vi "2020_day04.vi"() -> ()   [LabVIEW 2021]
uses:
  <vilib>/regexp/Match Regular Expression.xnode
panel:
  out "Task 2":i16
  out "Task 1":i16
  in  "Switch":bool caption="Ex. Data  vs.  User Data"
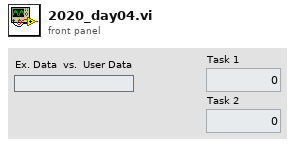
[diagram p1: front panel]
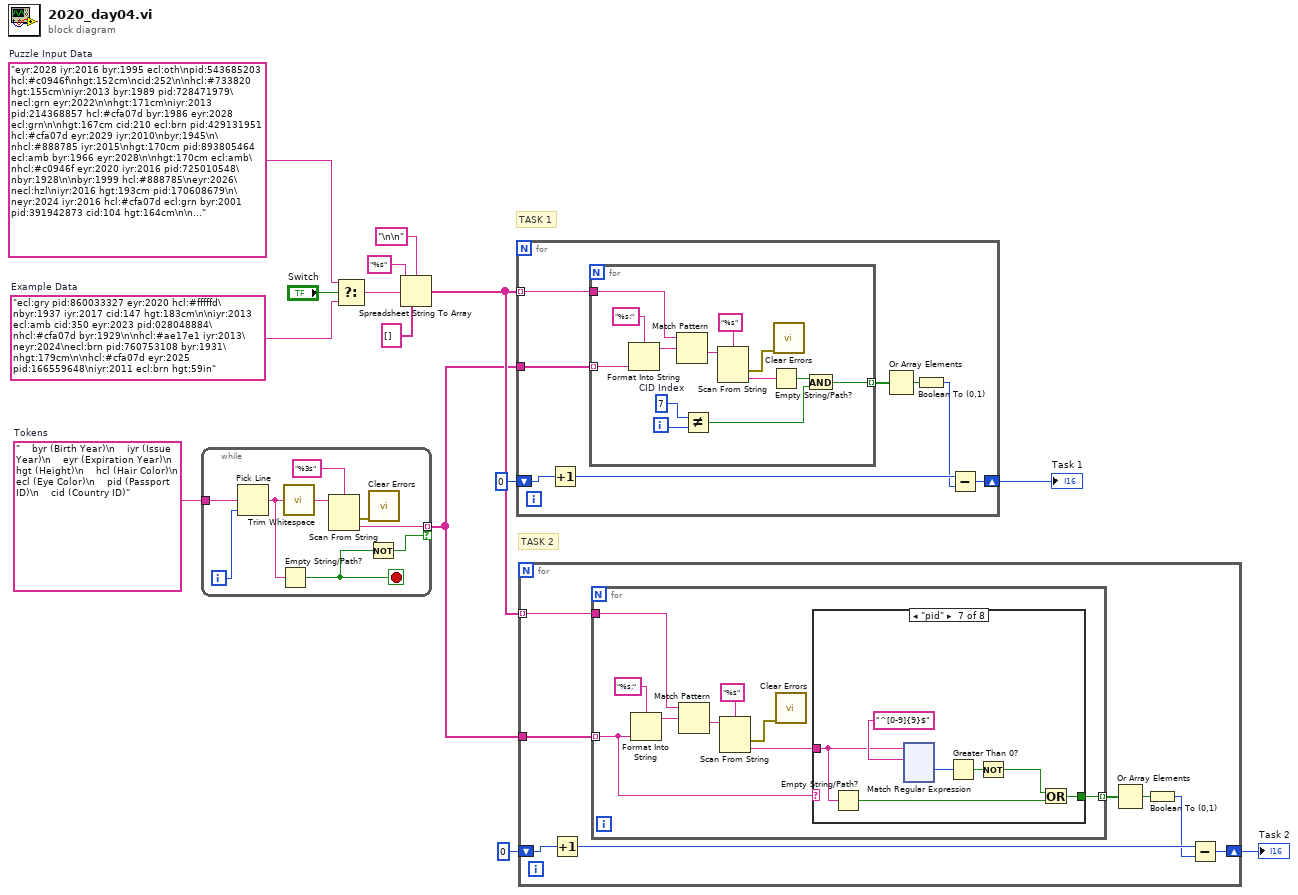
[diagram p0: block diagram]
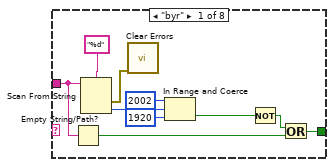
[diagram p2: hidden frame]
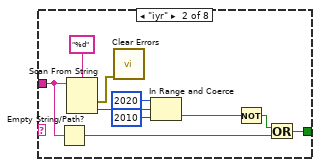
[diagram p3: hidden frame]
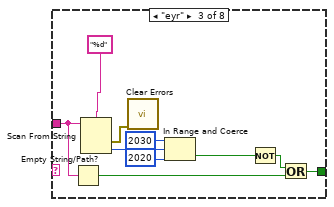
[diagram p4: hidden frame]
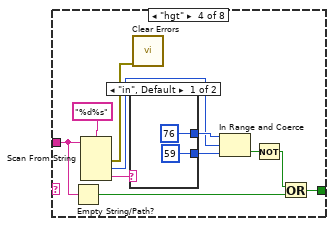
[diagram p5: hidden frame]
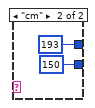
[diagram p6: hidden frame]
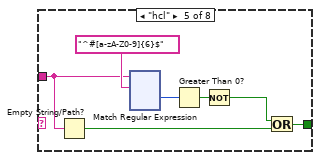
[diagram p7: hidden frame]
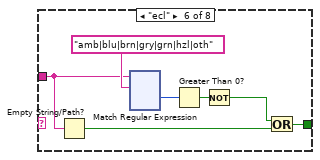
[diagram p8: hidden frame]
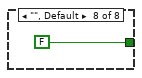
[diagram p9: hidden frame]
diagram:
  w7 = "    byr (Birth Year)\n    iyr (Issue Year)\n    eyr (Expiration Year)\n    hgt (Height)\n    hcl (Hair Color)\n    ecl (Eye Color)\n    pid (Passport ID)\n    cid (Country ID)"  # Tokens
  w12 = "eyr:2028 iyr:2016 byr:1995 ecl:oth\npid:543685203 hcl:#c0946f\nhgt:152cm\ncid:252\n\nhcl:#733820 hgt:155cm\niyr:2013 byr:1989 pid:728471979\necl:grn eyr:2022\n\nhgt:171cm\niyr:2013 pid:214368857 hcl:#cfa07d byr:1986 eyr:2028 ecl:grn\n\nhgt:167cm cid:210 ecl:brn pid:429131951 hcl:#cfa07d eyr:2029 iyr:2010\nbyr:1945\n\nhcl:#888785 iyr:2015\nhgt:170cm pid:893805464 ecl:amb byr:1966 eyr:2028\n\nhgt:170cm ecl:amb\nhcl:#c0946f eyr:2020 iyr:2016 pid:725010548\nbyr:1928\n\nbyr:1999 hcl:#888785\neyr:2026\necl:hzl\niyr:2016 hgt:193cm pid:170608679\n\neyr:2024 iyr:2016 hcl:#cfa07d ecl:grn byr:2001 pid:391942873 cid:104 hgt:164cm\n\niyr:2019\neyr:2025 pid:138912840 byr:1996\nhgt:166cm\nhcl:#888785 ecl:grn\n\niyr:2023 hcl:a58381 pid:#401a29 eyr:1940\nbyr:1920\necl:utc hgt:183cm\n\npid:493510244 ecl:gry hgt:153cm byr:1950 cid:181 eyr:2028\nhcl:#ceb3a1\niyr:2020\n\niyr:2018 pid:074340974 hgt:182cm\nhcl:#866857 byr:1988 ecl:hzl eyr:2023\n\nhcl:#866857 ecl:oth byr:1977 iyr:2014 hgt:180cm pid:860745884\neyr:2023\n\neyr:2026 pid:815594641\necl:gry iyr:2012 byr:1992 hgt:161cm hcl:#b6652a\n\necl:gry cid:338 eyr:2021 pid:777099878 hgt:193cm hcl:#efcc98\nbyr:1945\niyr:2015\n\niyr:2016 byr:1934 hcl:#b6652a\nhgt:162cm ecl:hzl\ncid:296\npid:742610207\neyr:2022\n\necl:#ba3242\nhgt:80 byr:1931\npid:550004054 iyr:1949 eyr:1944 hcl:fb3859\n\necl:amb eyr:2024\nbyr:1965 iyr:2010 pid:094059049\nhcl:#fffffd\nhgt:168cm\n\npid:159cm\niyr:1923 eyr:2032 hcl:701107 cid:343 ecl:gmt byr:2010\nhgt:177cm\n\neyr:2021\necl:grn byr:1991\nhcl:#fffffd hgt:167cm pid:243218792 iyr:2019\n\nhgt:157cm byr:2017 ecl:grn iyr:2012\neyr:2030 hcl:#18171d pid:173cm\n\npid:260101979 hgt:187cm eyr:2033 ecl:lzr\nbyr:2020 hcl:1058ce cid:133 iyr:2012\n\nhcl:#7d3b0c\npid:307828343 byr:2001\ncid:317 iyr:2013\neyr:2029\n\npid:472940417 eyr:1960\nhgt:181cm hcl:#c0946f cid:269\nbyr:2014\niyr:1956\n\nhcl:#18171d eyr:2021 byr:2001 pid:421443124\necl:brn iyr:2020 hgt:156cm\n\ncid:347 hgt:60in pid:359783692 byr:1932\necl:hzl\neyr:2023\nhcl:#888785 iyr:2019\n\npid:230915137\nbyr:1999\niyr:2011 eyr:2020 hcl:#7d3b0c ecl:hzl\nhgt:164cm\n\niyr:1989\nbyr:2008\nhgt:154cm\neyr:2028 pid:280298169\ncid:208\necl:oth\n\nbyr:1954 iyr:2017\necl:hzl\neyr:2026\npid:966957581 hgt:175cm hcl:#18171d\n\npid:308053355 hgt:192cm eyr:2022 ecl:amb cid:146 iyr:2015\nbyr:1991 hcl:#c0946f\n\nhcl:#a97842 pid:244441133 iyr:2019\nhgt:182cm\necl:amb cid:172 byr:1973 eyr:2029\n\niyr:2017\nbyr:1985 cid:215\necl:blu hcl:#623a2f hgt:160cm pid:157856689 eyr:2030\n\neyr:2027 ecl:#d72f9b hgt:162cm\niyr:2018 hcl:#a97842\nbyr:1945\npid:131243258\n\nhcl:#b3f2f0 pid:204254353 cid:169 eyr:2020\niyr:2013 hgt:172cm ecl:blu byr:1950\n\nbyr:1957 hcl:#c0946f hgt:152cm ecl:blu eyr:2027 pid:325917033\niyr:2010\n\necl:oth byr:1950 hgt:166cm pid:007352351\nhcl:#b6652a\niyr:2020\neyr:2024\n\nhgt:165 eyr:2030 iyr:2027\necl:#1a34f1 pid:2894591864 byr:2024 hcl:z\n\nbyr:1971 ecl:oth\nhgt:163cm eyr:2021 pid:040443396\n\nhgt:177cm\nbyr:1955 pid:585735590 iyr:2010 ecl:grn eyr:2024\nhcl:#602927\n\ncid:74\niyr:2010\npid:014378493 hgt:174cm eyr:2020\necl:grn byr:1944\n\npid:404141049\nbyr:1947 ecl:blu hgt:170cm iyr:2011\neyr:2028\nhcl:#cfa07d\n\necl:hzl byr:1938 pid:235085606 cid:180 hcl:8fb74c eyr:2021 hgt:73 iyr:2015\n\npid:860077423 ecl:gry\nhcl:#3e845b\nhgt:167cm byr:1933 iyr:2016 eyr:2021\n\nhcl:#733820 hgt:66in eyr:1920\necl:oth byr:1941 pid:979460474 iyr:2010\ncid:247\n\nhcl:#cfa07d ecl:#13bd36 hgt:193cm eyr:2027 pid:181cm byr:1952 iyr:1951\n\necl:brn hcl:#602927\nhgt:161cm\neyr:2027 pid:822749462 byr:1946\niyr:2014\n\nbyr:2013\niyr:2021 ecl:zzz eyr:2032 hgt:193in hcl:#a97842 pid:163cm\n\neyr:2029 cid:140\nbyr:1984\niyr:2018 hgt:187cm hcl:#b6652a pid:910674579\n\necl:hzl hgt:173cm pid:096026282\niyr:2014 byr:1956\neyr:2029 hcl:#866857\n\neyr:2024 iyr:2019 pid:301205967\ncid:276 byr:1957 hcl:#3fec29 ecl:gry hgt:165cm\n\niyr:2013 ecl:oth hgt:177cm hcl:#6b5442 eyr:2021 byr:1962 pid:006347857\n\necl:grt byr:1983 hcl:#cfa07d\nhgt:163cm\neyr:1979\niyr:1958 pid:796395720\n\niyr:2011 pid:415403544 hcl:#c0946f byr:1990 ecl:oth eyr:2023 hgt:73in\ncid:107\n\nhgt:166cm eyr:2029 iyr:2015\nhcl:#c0946f ecl:brn\nbyr:1964\npid:469449137\n\neyr:2023\nbyr:1969 iyr:2010 hgt:163cm hcl:#a97842 pid:570942274\necl:blu\n\nhcl:#623a2f\necl:brn hgt:183cm pid:524675399\neyr:2020 iyr:2012 byr:1981\n\niyr:2017 hcl:#fffffd eyr:2026\necl:gry byr:1979 hgt:152cm pid:505790864\n\nhgt:68in\nhcl:#c0946f iyr:2012\neyr:2023 pid:933562997 byr:1993\necl:grn\n\npid:267705171\nhgt:166cm byr:1970 iyr:2019 hcl:#341e13 ecl:oth\neyr:2030\n\necl:brn byr:1972 eyr:2026 pid:774637408 hgt:189cm iyr:2015 hcl:#341e13\n\nhgt:175cm eyr:2026 byr:2001 iyr:2020\nhcl:#733820 ecl:blu pid:686996160\n\nhgt:190cm hcl:#c0946f pid:228444464 byr:1987\niyr:2020 eyr:2030\necl:blu\n\nbyr:1990 hgt:179cm\npid:885359438 eyr:2028 iyr:2010 ecl:amb\nhcl:#67067e\n\nbyr:1945 hcl:#866857 eyr:2022 iyr:2019\npid:708146656 cid:65\nhgt:172cm ecl:brn\n\necl:hzl hgt:191cm\ncid:260 pid:010716679 iyr:2011 eyr:2029 byr:1920 hcl:#efcc98\n\niyr:2012\ncid:313 pid:264894705 byr:1951 hcl:#733820 eyr:2030 ecl:blu\nhgt:178cm\n\neyr:2027 pid:790510379\niyr:2013\necl:amb\nhgt:186cm\nhcl:#866857\nbyr:1926\n\npid:535750794 hgt:191cm iyr:2016 hcl:#a97842 eyr:2029\necl:hzl byr:1923\n\nbyr:2023 pid:#eb4c2a iyr:1939 ecl:grn hcl:06d729 hgt:73 eyr:2038\n\npid:792365221 iyr:2013 ecl:oth\nbyr:1997\nhgt:170cm hcl:#efcc98\neyr:2022\n\nhgt:192cm pid:874141668\nbyr:1957 iyr:2015\necl:gry\n\nhcl:#b6652a pid:770238761 eyr:2029 byr:1934 iyr:2013\necl:blu cid:177\nhgt:184cm\n\necl:hzl eyr:2024 hgt:72in pid:546439165\niyr:2013\nhcl:#c0946f cid:223 byr:1989\n\nbyr:1985\necl:utc pid:#ff1cbf\niyr:2018 hcl:#866857 hgt:169cm eyr:2026 cid:194\n\nhgt:189cm\neyr:2026 pid:120642045 ecl:blu\nhcl:#602927 cid:177\nbyr:1954 iyr:2012\n\npid:314624973\nbyr:1959 iyr:2015 hcl:#c0946f ecl:grn\neyr:2027 cid:349 hgt:156cm\n\nbyr:1978\niyr:2020 hgt:150cm cid:266 eyr:2026\npid:443912835 hcl:#b6652a\n\nhgt:174cm byr:1974 pid:729198828\necl:brn iyr:2014\nhcl:#18171d eyr:2027\n\npid:472891001 ecl:xry\nhgt:96 hcl:1b816a iyr:1954\nbyr:2015 eyr:2037\n\nbyr:1966 eyr:2022\niyr:2014\npid:848187688 hcl:#602927 ecl:gry hgt:152cm\n\nhgt:129 eyr:2037 cid:61 iyr:2009 byr:2027 hcl:#c0946f\npid:3569865\necl:#4e3d72\n\necl:gry\neyr:2021 pid:234525998 byr:1964 hgt:168cm cid:140\nhcl:#7d3b0c iyr:2013\n\necl:xry\ncid:86\nhgt:172in\nbyr:1972\niyr:2015 hcl:#7d3b0c pid:833809421 eyr:2030\n\npid:444365280 hgt:72in\necl:brn\nhcl:#b6652a byr:1985 eyr:2027 iyr:2012\n\niyr:2010 byr:2013 hgt:181cm eyr:2021\npid:072317444\necl:oth hcl:#866857\ncid:118\n\npid:4354408888 iyr:2012\nhcl:#b6652a cid:104\nhgt:96 eyr:2020\nbyr:1933 ecl:amb\n\neyr:2023 ecl:gry hcl:#a97842 pid:287719484 byr:1994\niyr:2011 hgt:163cm cid:299\n\nbyr:1932\nhgt:170cm\niyr:2014 pid:777844412 eyr:2040 hcl:#cfa07d ecl:brn\n\ncid:160 hgt:191cm eyr:2020 iyr:2012\necl:brn byr:1981 pid:077027782\n\ncid:182 hgt:176cm hcl:#7d3b0c\neyr:2030 ecl:blu pid:096742425 iyr:2010 byr:1963\n\nbyr:2010 cid:337 hcl:z pid:525126586 iyr:2010 hgt:73cm eyr:2040 ecl:blu\n\necl:gry\niyr:2017\nhgt:185cm hcl:#6b5442 byr:1993\neyr:2029 pid:366083139 cid:343\n\neyr:2028 ecl:amb\npid:878658841 byr:1960 hgt:179cm hcl:#18171d iyr:2010\n\npid:537309261 iyr:2015 hgt:187cm\nhcl:#4fe831 eyr:2026\necl:blu byr:1982\n\necl:brn hgt:163cm\neyr:2021 hcl:#6b5442 byr:1979 iyr:2013 pid:924759517\n\npid:683651053 hcl:#179c55\necl:blu byr:1989 hgt:190cm\niyr:2016\neyr:2030\n\necl:grn\niyr:2016 hcl:#b6652a\nbyr:1994 eyr:2020 pid:448424292 hgt:174cm\n\nhgt:157cm\necl:grn\nbyr:2000\npid:734707993 hcl:#341e13 iyr:2020\n\nhcl:#341e13 hgt:156cm iyr:2020 pid:299213638\nbyr:1947 ecl:hzl eyr:2023\n\nhgt:193cm hcl:#b6652a iyr:2014 ecl:hzl byr:1947 eyr:2025\npid:044486467\n\nbyr:1975\nhgt:159cm\necl:grn pid:318489576 eyr:2029 hcl:#6b5442\niyr:2020\n\niyr:2018 pid:512971930\nhcl:#888785 byr:1966 eyr:2024 hgt:158cm\ncid:100 ecl:gry\n\necl:amb eyr:2030 hgt:171cm hcl:#efcc98 pid:800921581 cid:339 byr:1980 iyr:2017\n\niyr:2019 cid:172\nhgt:152cm\neyr:2022 ecl:oth hcl:#602927 byr:1960\n\niyr:2019 pid:762312913\neyr:2029\necl:hzl\nhcl:#6b5442\nbyr:1940\nhgt:169cm cid:289\n\neyr:2022 ecl:gry byr:1976\niyr:2020 hcl:#733820 hgt:172cm pid:040331561\n\nhgt:171cm ecl:brn iyr:2013 eyr:2027 byr:1940 hcl:#a6e32a pid:223986941\n\nhcl:#341e13\neyr:2028 ecl:amb byr:1942\nhgt:166cm pid:435382099 iyr:2020\n\ncid:298 pid:641326891\nhgt:155cm hcl:#623a2f ecl:grn byr:1981 eyr:2025\niyr:2010\n\niyr:2015 pid:472000322 eyr:2021 byr:1977\necl:gry hgt:165cm cid:270\n\neyr:2027 byr:1956\npid:193087729 hcl:#ceb3a1\ncid:213 hgt:193cm ecl:oth\n\niyr:2014\nbyr:1971 cid:96\nhgt:74in\npid:136003336\neyr:2020 ecl:hzl hcl:#efcc98\n\nhcl:z pid:097595072 ecl:amb\niyr:2015 byr:2021\neyr:2039 hgt:188cm\n\npid:74823273\nhcl:#341e13\ncid:166 hgt:182cm byr:2026 iyr:2027 ecl:amb\neyr:2032\n\nbyr:1932 eyr:2022 pid:367248062 hgt:182cm ecl:oth hcl:#c0946f\niyr:2020\n\nhgt:72cm\niyr:2015 cid:234 byr:2013\necl:brn pid:9401866358\n\npid:022399779 iyr:2010 byr:1969 hcl:#6b5442\necl:grn eyr:2020\nhgt:189cm\n\nbyr:1971 iyr:2011 cid:161 ecl:brn hgt:153cm\neyr:2028 pid:819137905 hcl:#cfa07d\n\ncid:161 hgt:159cm iyr:2011 pid:815860793 hcl:#a97842 ecl:grn byr:1972 eyr:2027\n\necl:amb\nhgt:118 byr:1981 iyr:2019\nhcl:#a97842 eyr:2021 pid:270790642\n\nhcl:#b6652a pid:732272914 eyr:2030 hgt:183cm ecl:hzl\nbyr:1934\niyr:2018\n\neyr:2027\npid:877388498 hcl:#ceb3a1\nbyr:1925 cid:236 ecl:grn\niyr:2019 hgt:191cm\n\neyr:2020 ecl:brn hcl:#fffffd hgt:181cm pid:801311341 byr:1986 iyr:2010\n\nbyr:1925 cid:179 ecl:hzl pid:360641953 eyr:2030\nhgt:171in iyr:2015\nhcl:#602927\n\ncid:83 hgt:181cm\neyr:2028 byr:1941 pid:165937945 hcl:#888785 iyr:2014\necl:grn\n\nhcl:#a97842 byr:1928\niyr:2013\npid:870072019 hgt:76in\necl:oth cid:127 eyr:2026\n\ncid:169\nhgt:187cm pid:008180128 iyr:2013 byr:1991 hcl:#7d3b0c ecl:hzl eyr:2026\n\necl:amb\neyr:2027 hgt:155cm pid:586151564 iyr:2010\nbyr:1949\nhcl:#18171d\n\nhgt:167cm\niyr:2010 byr:1982 ecl:amb\ncid:235 pid:557737957 eyr:2020\nhcl:#ceb3a1\n\necl:grn byr:1939 hcl:#733820\neyr:2026 pid:993218958 iyr:2010\nhgt:150cm\n\nhgt:68in ecl:blu\nbyr:1965 iyr:2017 pid:854858050 eyr:2021\n\necl:gry pid:347763159 eyr:2024 iyr:2017 byr:1961\nhgt:151cm\nhcl:#623a2f\n\necl:utc hcl:#602927\npid:#1408ff byr:1941\ncid:82\niyr:2015 hgt:185cm eyr:2028\n\niyr:2020 hgt:151cm eyr:2025\nbyr:1934 hcl:#888785\npid:396545094 ecl:oth\n\nhgt:153cm\neyr:2028 hcl:#733820 ecl:gry iyr:2019\npid:081352630 byr:1943\n\neyr:2030\niyr:2011\necl:grn pid:313741119\nhgt:161cm byr:1946\nhcl:#a97842\n\nbyr:1968 ecl:gry\npid:742357550\neyr:2024 hcl:#18171d iyr:2018\nhgt:157cm\n\npid:387505919\necl:oth byr:1945\niyr:2014\nhgt:190cm hcl:#888785\neyr:2028\n\niyr:2017 hgt:175cm\nbyr:1989 eyr:2022\nhcl:#b6652a pid:499016802 ecl:gry cid:136\n\npid:490807331 iyr:2016\nhcl:#ceb3a1\nhgt:150cm eyr:2026\necl:amb byr:1967\n\niyr:2011\nhgt:155in\nhcl:#ceb3a1 pid:118497416\neyr:2029 byr:2011 ecl:oth\n\nhcl:03a888 byr:2029\necl:#6f7292 eyr:1969 iyr:2028 hgt:162cm pid:73551266\n\niyr:2016 hgt:182cm\nbyr:1966 ecl:grn eyr:2022\nhcl:#fffffd pid:061720787\n\nbyr:1971 hcl:z\neyr:2035 pid:158cm\necl:#d3ec19\n\nhcl:#623a2f hgt:156cm eyr:2028\necl:brn iyr:2013\nbyr:1980 pid:112283719\n\neyr:2020\nbyr:1956 iyr:2013\nhcl:#6b5442\necl:grn pid:876589775 hgt:179cm\n\nhgt:138\nbyr:2013 eyr:2040 iyr:2028 cid:197 ecl:#8844fd pid:8524414485\nhcl:z\n\neyr:2040\nhgt:173in hcl:z pid:#654654 byr:2016 iyr:2022 ecl:#452d22\n\niyr:2012 cid:265 eyr:2021 hgt:192cm\nbyr:1993 ecl:brn\n\neyr:2026 hcl:#888785\nhgt:158cm byr:1942\niyr:2015\necl:amb pid:546984106\n\niyr:2019\necl:hzl\nbyr:1922 eyr:2028 hgt:172cm\npid:465052232 hcl:#602927\n\npid:710362693 eyr:2023\nhcl:#c0946f byr:1951 ecl:grn\niyr:2019 hgt:190cm\n\niyr:2024 pid:#a08e69\nhcl:z byr:1966 ecl:#7b9978 eyr:2035\nhgt:69cm\n\nhcl:#efcc98\npid:164cm\niyr:2010 cid:194 hgt:71cm byr:1923 eyr:2026\n\nhgt:65in\niyr:2019 byr:1969 pid:466669360 eyr:2022 ecl:brn hcl:#b6652a\n\npid:42472559 hcl:#6f5763\neyr:2035\niyr:2014 hgt:154in byr:1939 ecl:grt cid:323\n\npid:715680334 hgt:166cm cid:283\nbyr:1982\niyr:2015 eyr:2030 hcl:#ceb3a1 ecl:grn\n\neyr:2018 iyr:2029\necl:brn\nbyr:2022 pid:#ff6df1\nhcl:z\nhgt:68cm\n\npid:094541122\neyr:2024 byr:1940\necl:amb iyr:2019 hgt:64in hcl:#733820\n\nhgt:163in\neyr:2022 ecl:utc hcl:#ceb3a1 iyr:2028\n\necl:gry pid:53552934\nhgt:193 byr:2021\neyr:2028\niyr:2011 cid:98 hcl:90c63f\n\neyr:2024 hcl:#cfa07d ecl:brn\niyr:2019 byr:1993 hgt:156cm pid:449484188\n\niyr:2020\nhgt:164cm hcl:#623a2f\npid:820731743 eyr:2025\nbyr:1997 ecl:hzl\n\nhcl:47242b ecl:utc hgt:156\npid:#9a9903 eyr:2030 iyr:1990\nbyr:2011\n\nhcl:#602927\nhgt:189cm\npid:949021883 iyr:2014 ecl:oth cid:327\neyr:2027 byr:1953\n\nhgt:189cm cid:301\nbyr:1982\necl:grn\neyr:2028 hcl:#733820 pid:796040143 iyr:2015\n\ncid:169 iyr:2013 pid:355177646 byr:1988\necl:oth\nhcl:#cfa07d\nhgt:185cm eyr:2022\n\npid:563150261 eyr:2020 ecl:brn byr:1996 hcl:#7d3b0c iyr:2018 hgt:189cm cid:84\n\ncid:188 eyr:2027\nbyr:1944\npid:486184923\niyr:2010 hgt:193cm hcl:#341e13 ecl:oth\n\niyr:2019\nbyr:1969 hgt:152cm pid:430698432 ecl:gry hcl:#888785 eyr:2026 cid:293\n\necl:gry\ncid:270 hcl:#602927 iyr:2017 hgt:151cm eyr:2029 pid:051398739 byr:1954\n\necl:oth eyr:2030 pid:024655030\nhgt:184cm byr:1969\nhcl:#18171d\n\neyr:2030\npid:899973263 hgt:178cm byr:1987 hcl:#cfa07d iyr:2012\necl:amb\n\niyr:1958 hgt:165cm pid:377677319\necl:grt eyr:2032 byr:2025\nhcl:bbfbe2\n\necl:blu\niyr:2016\nhgt:152cm byr:1964\nhcl:#c4f777\neyr:2021\npid:044307549 cid:80\n\necl:brn pid:330836320\nbyr:1963 cid:217 hgt:169cm\neyr:2024\niyr:2019 hcl:#ceb3a1\n\nbyr:1976 eyr:2027\npid:452662874 hgt:192cm ecl:oth iyr:2018 hcl:#602927\n\neyr:2027 hgt:183cm ecl:brn iyr:2017 hcl:#341e13 pid:827463598\n\necl:brn pid:930667228 cid:310 iyr:2020\neyr:2027 hgt:160cm byr:1932 hcl:#c0946f\n\npid:955804028 byr:1983\nhcl:#fffffd\nhgt:178cm iyr:2013\neyr:2021 ecl:gry\n\nhgt:189cm eyr:2021 pid:430243363 iyr:2015 hcl:#ceb3a1\nbyr:2000 ecl:oth cid:284\n\npid:436671537 hcl:#cfa07d iyr:2011 cid:106 hgt:171cm\necl:blu eyr:2021 byr:1943\n\neyr:2028 hgt:169cm\niyr:2015 pid:177443573 byr:1945\nhcl:#c0946f ecl:gry\n\nhcl:#fffffd byr:1995 eyr:2021\necl:grn\nhgt:192cm iyr:2010 pid:754912745\n\npid:330882171 iyr:2015 cid:211 ecl:grn byr:1961 eyr:2021 hcl:z\nhgt:169cm\n\nbyr:1926 eyr:2029 pid:178633665 cid:141 iyr:2017 hcl:#b99eb9\nhgt:178cm ecl:brn\n\neyr:2022 ecl:hzl hcl:#cfa07d hgt:168cm iyr:2015\nbyr:1982 pid:645675448\n\necl:blu byr:1980 hgt:186cm iyr:2010 cid:94 hcl:#c0946f eyr:2027 pid:384440210\n\ncid:309 hcl:#602927 hgt:192cm eyr:2027 ecl:amb\npid:527932745 iyr:2012 byr:1982\n\ncid:132\necl:blu iyr:2016\neyr:2027 byr:1940 hcl:#341e13 hgt:166cm pid:613386501\n\npid:360563823 eyr:2028 byr:1990 iyr:2016\necl:blu cid:287 hgt:162cm hcl:#888785\n\nhgt:161cm\nbyr:2002\nhcl:#623a2f pid:535361632\necl:gry eyr:2021 iyr:2013\n\nhgt:67in\nbyr:1967\ncid:333 hcl:#cfa07d\niyr:2012 eyr:2024 ecl:hzl pid:538161833\n\necl:#2bc145 eyr:1963 iyr:2030\ncid:241 hcl:2fc384 hgt:156in pid:2899917140\nbyr:2005\n\neyr:2021 pid:021590229 ecl:gry\nhgt:164cm iyr:2013 hcl:#efcc98 byr:1985\n\necl:hzl byr:1943\ncid:279 pid:979130395\niyr:2011\nhgt:165cm\neyr:2021\nhcl:#f331b3\n\nhgt:161cm\nhcl:#888785 byr:1981 pid:835477382 eyr:2025 iyr:2012\ncid:348\necl:blu\n\nhgt:159cm hcl:b4ce6a cid:319 eyr:2035 iyr:1965 ecl:oth\nbyr:2010 pid:158cm\n\niyr:2020\neyr:2026 ecl:grn hcl:#a97842 pid:126915503\nhgt:178cm byr:1986\n\nhgt:184cm ecl:hzl\ncid:67 iyr:2020 eyr:2026 pid:168775568 byr:1944 hcl:#a97842\n\nhcl:#fffffd iyr:2016 pid:379463363\necl:oth\nhgt:179cm byr:1988\neyr:2028\n\nhcl:#cfa07d ecl:amb eyr:2030 pid:320360020\niyr:2016 hgt:172cm byr:1961\n\ncid:221 hcl:#cfa07d byr:1946 eyr:2024 ecl:oth pid:066950409 hgt:173cm\niyr:2020\n\nhcl:#602927 eyr:2028 ecl:gry iyr:2019 pid:583204134 byr:1966 hgt:178cm\n\nbyr:1930\niyr:2020 ecl:hzl\nhcl:#ceb3a1 pid:285751767 cid:287 eyr:2023 hgt:192cm\n\neyr:2024\necl:hzl cid:87 iyr:2015\nhgt:152cm hcl:#18171d pid:959574669\nbyr:1990\n\npid:45938863\nhcl:49c7ce cid:349 hgt:181cm\neyr:2023 ecl:grn iyr:2015 byr:1948\n\nhcl:#866857 iyr:2012 ecl:amb cid:132 byr:1955 hgt:162cm pid:597748286 eyr:2023\n\npid:293364535 byr:2024\nhgt:177cm eyr:2039\niyr:2020 hcl:#dae928 ecl:hzl\n\npid:212659709 iyr:2018\nhgt:188cm\nhcl:#efcc98 byr:1974 eyr:2029 ecl:oth cid:244\n\ncid:140\necl:amb\neyr:2022 hgt:181cm hcl:#efcc98\nbyr:1943\niyr:2016\n\ncid:71 hgt:151cm pid:5063555219 eyr:2023 ecl:hzl\nbyr:2019\nhcl:#7d3b0c iyr:2023\n\nhgt:157in pid:#298b06 iyr:2030 ecl:#66a631 eyr:2035 hcl:z byr:2019\n\nhgt:190cm iyr:1943\npid:644021656 hcl:#6b621c\necl:oth eyr:2021 byr:1923\n\necl:hzl iyr:2012 eyr:2023 pid:881271720 hcl:#ceb3a1 hgt:172cm\nbyr:1957\n\niyr:2017 hcl:#888785\necl:amb hgt:170cm byr:1967 pid:198856675 eyr:2027\n\neyr:2026\necl:gry\npid:834980363 hcl:#733820 byr:1930\nhgt:175cm iyr:2018\ncid:214\n\nhcl:#efcc98 eyr:2029 iyr:2010 pid:980087545\necl:brn hgt:157cm\n\npid:57513658 iyr:2011 byr:1993 ecl:brn eyr:2027 hcl:#6b5442 hgt:165cm\n\necl:hzl\neyr:2025\nhcl:#733820\nhgt:169cm iyr:2018 cid:328 byr:1999 pid:694719489\n\neyr:2023\ncid:125 byr:1925\nhgt:185cm pid:806769540 iyr:2013 ecl:hzl\nhcl:#866857\n\niyr:2010 cid:225\necl:hzl eyr:2027 pid:615545523\nhcl:#733820\nbyr:1994\nhgt:166cm\n\nbyr:1941 ecl:gry iyr:2019 eyr:2026 hgt:73cm hcl:#602927\npid:352996721\n\npid:140250433\neyr:2030 ecl:grn\nhcl:#fffffd iyr:2011 byr:1937 hgt:185cm\n\necl:gry byr:2002 iyr:2017 hcl:#b6652a cid:261 pid:178cm eyr:2022 hgt:166cm\n\necl:grn iyr:2010 eyr:2022 byr:1924\npid:214641920 hcl:#ceb3a1\nhgt:155cm\n\nhcl:z pid:150cm ecl:utc iyr:1981\neyr:2034\nhgt:156in cid:260 byr:2027\n\nbyr:1987 hgt:66in\neyr:2021 pid:876757018 iyr:2015 hcl:d596e4 ecl:hzl\n\ncid:116 ecl:oth hgt:180cm\niyr:2020 byr:1942 hcl:#2fc31f\neyr:2027\npid:253569416\n\npid:509387921\neyr:2022\nhcl:#888785 ecl:oth hgt:193cm\niyr:2012 cid:97\nbyr:1975\n\nhcl:#18171d hgt:190cm pid:062827417 byr:1939\niyr:2019 eyr:2022\necl:hzl\n\niyr:2025\nbyr:2028\nhgt:165in eyr:2027 pid:6259332452\nhcl:#478251\n\niyr:2018 eyr:2026 pid:523863237\nhgt:187cm\necl:oth\nbyr:1944\nhcl:#a97842\n\nhgt:181cm hcl:#733820 pid:923996316\ncid:110\niyr:2011 byr:1949 ecl:blu eyr:2023\n\npid:304792392 hcl:487823 eyr:2020\nhgt:70cm byr:2024\niyr:1953\necl:blu\n\npid:142200694\necl:oth hcl:#888785 eyr:2028\nhgt:152cm byr:1954 iyr:2018\n\necl:utc\niyr:2015 byr:1932 hcl:#623a2f\neyr:2027 hgt:183cm pid:036300444\n\niyr:2014 ecl:hzl byr:1935 hgt:190cm hcl:#efcc98 pid:945893288\neyr:2025\n\nhcl:#efcc98 pid:252639104 hgt:188cm\nbyr:1998 iyr:2019 ecl:grn\neyr:2023\n\nhcl:58aa4a byr:1930 hgt:193cm\niyr:1998 cid:196 ecl:brn\neyr:2032\n\niyr:2015 ecl:hzl\nhgt:193cm pid:653794674 eyr:2024\nhcl:#fffffd byr:1921\n\npid:980680460 byr:1962 ecl:blu\niyr:2013\nhcl:#72cace\neyr:2030\nhgt:180cm\n\neyr:2025\nhgt:182cm hcl:#ceb3a1 iyr:2010 byr:1945 cid:314 pid:597769706 ecl:amb\n\npid:761757504\nhcl:#888785 hgt:161cm iyr:2015\nbyr:1939 eyr:2025\ncid:326 ecl:blu\n\necl:gry\nhgt:163cm byr:1981\npid:330818500 iyr:2017 eyr:2024\ncid:71 hcl:#888785\n\npid:190cm cid:267 iyr:2015 ecl:brn\nhcl:869252\nbyr:1935 hgt:142 eyr:2033\n\ncid:239\neyr:2038 ecl:lzr hcl:z iyr:1987 pid:4632768239\nhgt:162in\n\npid:158038227 ecl:brn byr:1995 eyr:2028 hcl:#efcc98\ncid:252 iyr:2021\nhgt:184cm\n\neyr:2027\ncid:124 ecl:amb hgt:165cm byr:1949\npid:727126101 iyr:2010 hcl:#602927\n\necl:grn\nbyr:1966 pid:184245393 hgt:164cm\neyr:2022\niyr:2014 hcl:#866857\n\ncid:62 hgt:180cm eyr:2027 hcl:#18171d\niyr:2017 ecl:blu byr:1942 pid:930210027\n\necl:grn hgt:171cm iyr:2017 hcl:#fffffd eyr:2029 byr:1946 pid:863414762\ncid:95\n\neyr:2025 ecl:grn iyr:2019 cid:226 hcl:#b6652a\nbyr:1932 pid:715708549\nhgt:156cm\n\npid:505158338 iyr:2019 byr:1981 hgt:193cm\nhcl:#696a5c cid:57 ecl:hzl eyr:2023\n\nbyr:1987\nhgt:155cm cid:99 ecl:grn iyr:2010\nhcl:#c0946f eyr:2023\npid:431067921\n\nhgt:190in\nhcl:z eyr:2029 pid:74228790\niyr:2016 byr:2018 ecl:brn\n\neyr:2022\necl:xry hgt:154cm pid:62205162\niyr:2014 byr:1936\ncid:61\n\necl:amb eyr:2026\nbyr:1966 cid:95 hcl:#733820 pid:957767251 iyr:2013 hgt:157cm\n\nbyr:1969\nhgt:156cm iyr:2013 ecl:blu hcl:#a97842\ncid:183\npid:960672229 eyr:2020\n\niyr:2013\ncid:243 eyr:2028 hgt:192cm hcl:#efcc98\necl:grn pid:222407433 byr:1978\n\niyr:2014 byr:1935\neyr:2021 cid:235 pid:#1b34e1\nhcl:#89313f hgt:164cm ecl:blu\n\necl:hzl iyr:2016 cid:327\nbyr:1923 pid:695935353 hgt:184cm\nhcl:#a97842\neyr:2028\n\npid:6010745668\nbyr:1934 ecl:oth eyr:2020 hgt:164cm\nhcl:#733820\niyr:2016\n\necl:blu pid:071991002 eyr:2021 byr:1978 cid:321\nhcl:#efcc98\niyr:2013 hgt:68in\n\necl:grn iyr:2015 pid:137792524 cid:156\nhcl:#efcc98\neyr:2029 byr:1955\nhgt:165cm\n\nbyr:1949\nhgt:176cm pid:531868428\nhcl:#cfa07d ecl:brn iyr:2014 eyr:2024\n\niyr:1955 cid:108 pid:712137140 byr:2019 eyr:2040 hgt:184cm hcl:220cfe ecl:#551592\n\niyr:2016 eyr:2030\nhgt:177cm cid:137 ecl:brn\nhcl:#efcc98 pid:712202745 byr:1938\n\npid:357180007 iyr:2010 ecl:grn\nbyr:1991\nhcl:#341e13\neyr:2020 hgt:159cm\n\neyr:2023 ecl:grn\nhcl:#733820 iyr:2020 byr:1927 hgt:151cm\npid:165936826\n\necl:gry\npid:794227261 iyr:2014 eyr:2030\nhcl:#18171d\nbyr:1994\nhgt:162cm\n\niyr:2017 eyr:2024\nhcl:#7d3b0c cid:279\necl:gry byr:1981 hgt:176cm pid:973822115\n\neyr:2029\nhgt:152cm hcl:#fffffd ecl:amb byr:1946 iyr:2013\ncid:62 pid:005240023\n\niyr:2010\necl:amb hcl:#341e13 hgt:184cm\neyr:2027\npid:976217816 byr:1950\n\necl:grn hgt:178cm cid:192 hcl:#602927 pid:684333017 eyr:2022\niyr:2011 byr:1987\n\npid:306960973 ecl:hzl hgt:168cm\nbyr:1954 iyr:2015 eyr:2029 hcl:#602927\n\nhcl:#18171d\nbyr:1973 ecl:hzl hgt:174cm pid:922891164\niyr:2013\neyr:2023\n\nbyr:1998 hgt:189cm pid:472066200 ecl:gry iyr:2012 eyr:2021 hcl:#c0946f cid:299\n\niyr:2014\neyr:2028 byr:1922 pid:594856217 hgt:158cm\necl:oth\nhcl:#623a2f\n\npid:215206381 byr:1928\nhgt:163cm\nhcl:#b6652a ecl:oth iyr:2011\n\ncid:145 iyr:2013\necl:#38a290\neyr:2034\nhcl:#602927 hgt:186cm pid:517498756\nbyr:1945\n\nhcl:#5637d2 eyr:2030 byr:1955\nhgt:187cm\npid:862655087 iyr:2014 ecl:grn\n\nhcl:#7d3b0c hgt:176cm iyr:2019\neyr:2029 byr:1980 ecl:hzl\ncid:346 pid:703908707\n\nhgt:185cm\niyr:2017\ncid:120 eyr:2020 hcl:#733820 ecl:blu pid:458522542 byr:1966\n\npid:#725759\nhcl:#602927 iyr:2013 byr:2003 eyr:2023 cid:100"  # Puzzle Input Data
  w13 = "ecl:gry pid:860033327 eyr:2020 hcl:#fffffd\nbyr:1937 iyr:2017 cid:147 hgt:183cm\n\niyr:2013 ecl:amb cid:350 eyr:2023 pid:028048884\nhcl:#cfa07d byr:1929\n\nhcl:#ae17e1 iyr:2013\neyr:2024\necl:brn pid:760753108 byr:1931\nhgt:179cm\n\nhcl:#cfa07d eyr:2025 pid:166559648\niyr:2011 ecl:brn hgt:59in"  # Example Data
  # "TASK 2"
  # "TASK 1"
  n1 = while {
    tunnel: w7 -> [w23]
    tunnel: [w18] -> w1 mode=indexing if=w17
    i -> [w22]
    stop <- w16 stop-if-true
    n2 = Pick Line(multi-line string=w23, line index=w22) -> (output string=w21:string)  [unwired: 1 in]
    n3 = Empty String/Path?(string/path=w21) -> (empty?=w16:bool)
    n4 = call <vilib>:"Trim Whitespace.vi"("string"=w21) -> ("trimmed string"=w20:string)  [unwired: 1 in]
    n5 = Scan From String(format string="%3s", input string=w20) -> (error out=w15:errorcluster, output 1=w18:string)  [unwired: 3 in, 2 out]
    n6 = Not(x=w16) -> (.not. x?=w17:bool)
    n7 = call <vilib>:"Clear Errors.vi"("error in (no error)"=w15) -> ()  [unwired: 5 in, 2 out]
  }
  n8 = Select(t=w12, s="Switch", f=w13) -> (s? t:f=w11:string)
  n9 = Spreadsheet String To Array(delimiter (Tab)="\n\n", format string="%s", spreadsheet string=w11, array type (2D Dbl)=string[] []) -> (array=w2:string[])
  n10 = for {
    tunnel: w2 -> [w30] mode=indexing
    tunnel: w1 -> [w31]
    shift-right: [w25] -> w5
    shift-left: i16 0 -> [w24]
    n11 = Increment(x=w24) -> (x+1=w27:i16)
    n12 = for {
      tunnel: w31 -> [w44] mode=indexing
      tunnel: w30 -> [w42]
      tunnel: [w32] -> w29 mode=indexing
      i -> [w36]
      w35 = 7  # CID Index
      n13 = Format Into String(format string="%s:", w44) -> (resulting string=w41:string)  [unwired: 2 in, 1 out]
      n14 = Match Pattern(string=w42, regular expression=w41) -> (after substring=w40:string)  [unwired: 1 in, 3 out]
      n15 = Not Equal?(x=w35, y=w36) -> (x != y?=w33:bool)
      n16 = Scan From String(format string="%s", input string=w40) -> (error out=w38:errorcluster, output 1=w37:string)  [unwired: 3 in, 2 out]
      n17 = Empty String/Path?(string/path=w37) -> (empty?=w34:bool)
      n18 = call <vilib>:"Clear Errors.vi"("error in (no error)"=w38) -> ()  [unwired: 5 in, 2 out]
      n19 = And(x=w34, y=w33) -> (x .and. y?=w32:bool)
    }
    n20 = Or Array Elements(Boolean array=w29) -> (logical OR=w28:bool)
    n21 = Boolean To (0,1)(Boolean=w28) -> (0, 1=w26:i16)
    n22 = Subtract(x=w27, y=w26) -> (x-y=w25:i16)
  }
  "Task 1" <- w5
  n23 = for {
    tunnel: w2 -> [w51] mode=indexing
    tunnel: w1 -> [w52]
    shift-right: [w49] -> w4
    shift-left: i16 0 -> [w48]
    n24 = Increment(x=w48) -> (x+1=w50:i16)
    n25 = for {
      tunnel: w52 -> [w54] mode=indexing
      tunnel: w51 -> [w60]
      tunnel: [w53] -> w46 mode=indexing
      n26 = Format Into String(format string="%s:", w54) -> (resulting string=w59:string)  [unwired: 2 in, 1 out]
      n27 = Match Pattern(string=w60, regular expression=w59) -> (after substring=w58:string)  [unwired: 1 in, 3 out]
      n28 = Scan From String(format string="%s", input string=w58) -> (error out=w56:errorcluster, output 1=w55:string)  [unwired: 3 in, 2 out]
      n29 = call <vilib>:"Clear Errors.vi"("error in (no error)"=w56) -> ()  [unwired: 5 in, 2 out]
      n30 = case shown="\"pid\"" w54 {
        tunnel: w55 -> [w71 w81 w91 w102 w109 w233 w357 _]
        tunnel: [w63 w73 w83 w99 w112 w236 w360 FALSE] -> w53
        frame "byr" {
          n31 = Empty String/Path?(string/path=w71) -> (empty?=w64:bool)
          n32 = Scan From String(format string="%d", input string=w71) -> (error out=w62:errorcluster, output 1=w69:i32)  [unwired: 3 in, 2 out]
          n33 = call <vilib>:"Clear Errors.vi"("error in (no error)"=w62) -> ()  [unwired: 5 in, 2 out]
          n34 = In Range and Coerce(upper limit=2002, x=w69, lower limit=1920) -> (In Range?=w66:bool)  [unwired: 1 out]
          n35 = Not(x=w66) -> (.not. x?=w65:bool)
          n36 = Or(x=w65, y=w64) -> (x .or. y?=w63:bool)
        }
        frame "iyr" {
          n37 = Empty String/Path?(string/path=w81) -> (empty?=w74:bool)
          n38 = Scan From String(format string="%d", input string=w81) -> (error out=w72:errorcluster, output 1=w79:i32)  [unwired: 3 in, 2 out]
          n39 = call <vilib>:"Clear Errors.vi"("error in (no error)"=w72) -> ()  [unwired: 5 in, 2 out]
          n40 = In Range and Coerce(upper limit=2020, x=w79, lower limit=2010) -> (In Range?=w76:bool)  [unwired: 1 out]
          n41 = Not(x=w76) -> (.not. x?=w75:bool)
          n42 = Or(x=w75, y=w74) -> (x .or. y?=w73:bool)
        }
        frame "eyr" {
          n43 = Empty String/Path?(string/path=w91) -> (empty?=w84:bool)
          n44 = Scan From String(format string="%d", input string=w91) -> (error out=w82:errorcluster, output 1=w89:i32)  [unwired: 3 in, 2 out]
          n45 = call <vilib>:"Clear Errors.vi"("error in (no error)"=w82) -> ()  [unwired: 5 in, 2 out]
          n46 = In Range and Coerce(upper limit=2030, x=w89, lower limit=2020) -> (In Range?=w86:bool)  [unwired: 1 out]
          n47 = Not(x=w86) -> (.not. x?=w85:bool)
          n48 = Or(x=w85, y=w84) -> (x .or. y?=w83:bool)
        }
        frame "hgt" {
          n49 = Empty String/Path?(string/path=w102) -> (empty?=w100:bool)
          n50 = Scan From String(format string="%d%s", input string=w102) -> (error out=w98:errorcluster, output 1=w94:i32, output 2=w97:string)  [unwired: 4 in, 2 out]
          n51 = case shown="\"in\", Default" w97 {
            tunnel: [59 ("lower limit") 150 ("lower limit")] -> w96
            tunnel: [76 ("upper limit") 193 ("upper limit")] -> w95
            frame "in", Default {
            }
            frame "cm" {
            }
          }
          n52 = call <vilib>:"Clear Errors.vi"("error in (no error)"=w98) -> ()  [unwired: 5 in, 2 out]
          n53 = In Range and Coerce(upper limit=w95, x=w94, lower limit=w96) -> (In Range?=w93:bool)  [unwired: 1 out]
          n54 = Not(x=w93) -> (.not. x?=w92:bool)
          n55 = Or(x=w92, y=w100) -> (x .or. y?=w99:bool)
        }
        frame "hcl" {
          n56 = Empty String/Path?(string/path=w109) -> (empty?=w111:bool)
          n57 = xnode "Match Regular Expression"("input string"=w109, "regular expression"="^#[a-zA-Z0-9]{6}$") -> ("offset past match"=w108:i32)  [unwired: 4 in, 4 out]
          n58 = Greater Than 0?(x=w108) -> (x > 0?=w107:bool)
          n59 = Not(x=w107) -> (.not. x?=w113:bool)
          n60 = Or(x=w113, y=w111) -> (x .or. y?=w112:bool)
        }
        frame "ecl" {
          n61 = Empty String/Path?(string/path=w233) -> (empty?=w235:bool)
          n62 = xnode "Match Regular Expression"("input string"=w233, "regular expression"="amb|blu|brn|gry|grn|hzl|oth") -> ("offset past match"=w232:i32)  [unwired: 4 in, 4 out]
          n63 = Greater Than 0?(x=w232) -> (x > 0?=w231:bool)
          n64 = Not(x=w231) -> (.not. x?=w237:bool)
          n65 = Or(x=w237, y=w235) -> (x .or. y?=w236:bool)
        }
        frame "pid" {
          n66 = Empty String/Path?(string/path=w357) -> (empty?=w359:bool)
          n67 = xnode "Match Regular Expression"("input string"=w357, "regular expression"="^[0-9]{9}$") -> ("offset past match"=w356:i32)  [unwired: 4 in, 4 out]
          n68 = Greater Than 0?(x=w356) -> (x > 0?=w355:bool)
          n69 = Not(x=w355) -> (.not. x?=w361:bool)
          n70 = Or(x=w361, y=w359) -> (x .or. y?=w360:bool)
        }
        frame "", Default {
        }
      }
    }
    n71 = Or Array Elements(Boolean array=w46) -> (logical OR=w47:bool)
    n72 = Boolean To (0,1)(Boolean=w47) -> (0, 1=w45:i16)
    n73 = Subtract(x=w50, y=w45) -> (x-y=w49:i16)
  }
  "Task 2" <- w4
